vi "Pcre2Config8.vi"(8 "error in":errorcluster, 11 "What":u32) -> (0 "error out":errorcluster, 2 "String":string, 3 "Info":u32)   [LabVIEW 2021, in "libpcre2-8.lvlib"]
uses:
  libpcre2-8.lvlib
  libpcre2-8-x32.dll
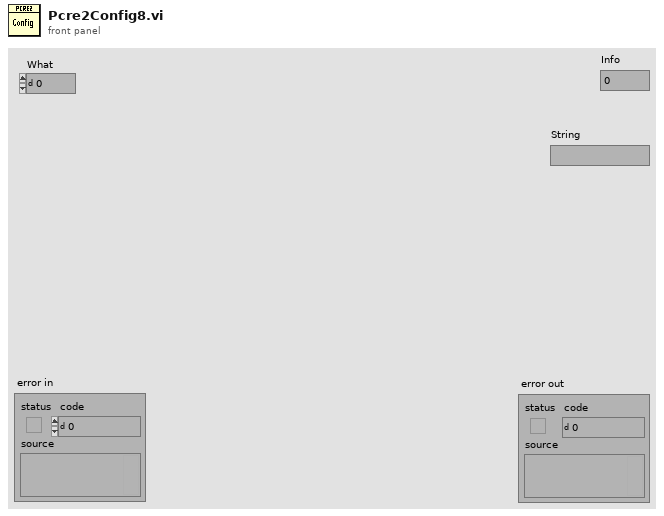
[diagram p1: front panel]
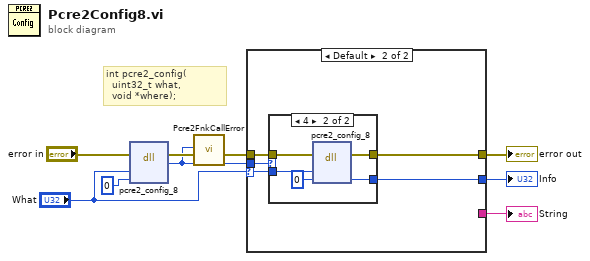
[diagram p0: block diagram]
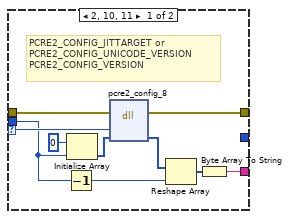
[diagram p2: hidden frame]
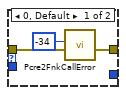
[diagram p3: hidden frame]
diagram:
  # "int pcre2_config(\n  uint32_t what,\n  void *where);"
  n1 = dll-call lib="libpcre2-8-x*.dll" fn="pcre2_config_8"(error in="error in", "what"="What", "where"=u64 0) -> (error out=w7:errorcluster, "return type"=w5:i32)  [unwired: 4 in, 1 out]
  n2 = call "Pcre2FnkCallError.vi"("error in"=w7, "ErrorCode"=w5) -> ("error out"=w6:errorcluster)  [unwired: 9 in]
  n3 = case shown="Default" "What" {
    selector: "What" -> [w16 w23]
    tunnel: w6 -> [w19 w24]
    tunnel: [w18 w21] -> w2
    tunnel: w5 -> [w12 w20]
    tunnel: [w13 _] -> w4
    tunnel: [_ w22] -> w3
    frame 2, 10, 11 {
      # "PCRE2_CONFIG_JITTARGET or\nPCRE2_CONFIG_UNICODE_VERSION\nPCRE2_CONFIG_VERSION"
      n4 = Decrement(x=w12) -> (x-1=w11:i32)
      n5 = Initialize Array(u8 0 ("U8"), w12) -> (w17:u8[])
      n6 = dll-call lib="libpcre2-8-x*.dll" fn="pcre2_config_8"(error in=w19, "what"=w16, "where"=w17) -> (error out=w18:errorcluster, "where"=w15:u8[])  [unwired: 4 in, 1 out]
      n7 = Reshape Array(w15, w11) -> (w14:u8[])
      n8 = Byte Array To String(unsigned byte array=w14) -> (string=w13:string)
    }
    frame Default {
      n9 = case shown="4" w20 {
        tunnel: w24 -> [w27 w32]
        tunnel: w23 -> [_ w31]
        tunnel: [_ w29] -> w22
        tunnel: [w26 w28] -> w21
        frame 0, Default {
          n10 = call "Pcre2FnkCallError.vi"("error in"=w27, "ErrorCode"=-34) -> ("error out"=w26:errorcluster)  [unwired: 9 in]
        }
        frame 4 {
          n11 = dll-call lib="libpcre2-8-x*.dll" fn="pcre2_config_8"(error in=w32, "what"=w31, "where"=u32 0) -> (error out=w28:errorcluster, "where"=w29:u32)  [unwired: 4 in, 1 out]
        }
      }
    }
  }
  "error out" <- w2
  "Info" <- w3
  "String" <- w4
